vi "set_raw_channels.vi"(8 "error in (no error)":errorcluster, 10 "raw channels":refnum<class "Image.lvclass">[](array[class]), 11 "DL090211ImageAssemblerScaffold.lvclass in":refnum<class "ImageAssemblerDL090211Scaffold.lvclass">) -> (0 "error out":errorcluster, 3 "DL090211ImageAssemblerScaffold.lvclass out":refnum<class "ImageAssemblerDL090211Scaffold.lvclass">)   [LabVIEW 2010, in "ImageAssemblerDL090211Scaffold.lvclass"]
uses:
  ImageAssemblerDL090211Scaffold.lvclass
  common/classes/Image/Image/Image.lvclass
  ImageAssemblerDL090211Scaffold.lvclass/ImageAssemblerDL090211Scaffold.ctl
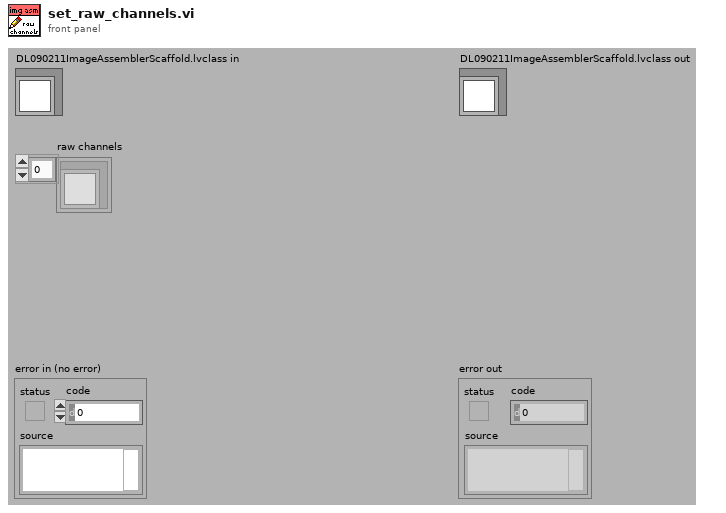
[diagram p1: front panel]
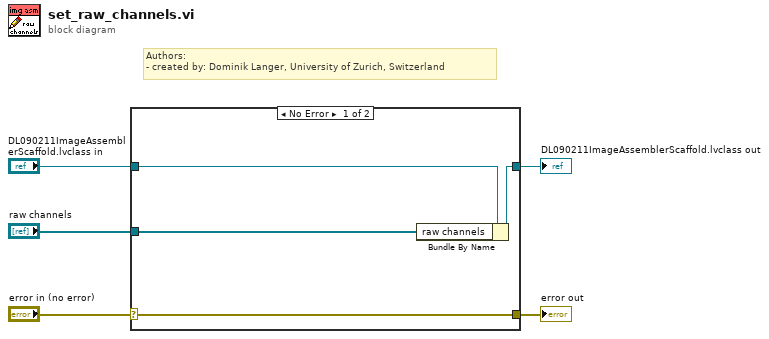
[diagram p0: block diagram]
diagram:
  # "Authors: \n- created by: Dominik Langer, University of Zurich, Switzerland"
  n1 = case shown="No Error" "error in (no error)" {
    selector: "error in (no error)" -> [w9 w10]
    tunnel: [w9 w10] -> w4
    tunnel: [w7 w11] -> w2
    tunnel: "DL090211ImageAssemblerScaffold.lvclass in" -> [w8 w11]
    tunnel: "raw channels" -> [w6 _]
    frame No Error {
      n2 = Bundle By Name(cluster=w8, "raw channels"=w6) -> (w7:refnum<class "ImageAssemblerDL090211Scaffold.lvclass">)
    }
    frame Error {
    }
  }
  "error out" <- w4
  "DL090211ImageAssemblerScaffold.lvclass out" <- w2
